vi "Rescale.vi"(8 "Error In":errorcluster, 11 "Pane Relief Main UI in":refnum<class "Pane Relief Main UI.lvclass">) -> (0 "Error Out":errorcluster, 3 "Pane Relief Main UI out":refnum<class "Pane Relief Main UI.lvclass">)   [LabVIEW 2017, in "Pane Relief Main UI.lvlib" / "Pane Relief Main UI.lvclass"]
uses:
  Pane Relief Main UI.lvclass
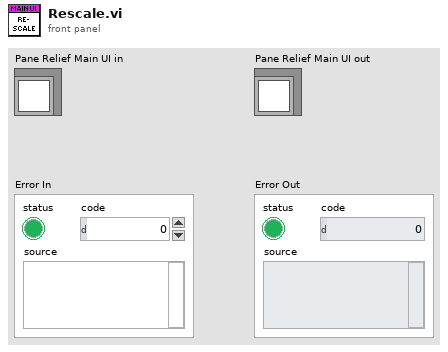
[diagram p1: front panel]
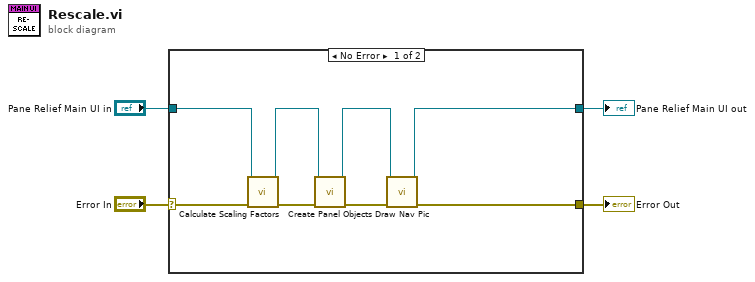
[diagram p0: block diagram]
diagram:
  n1 = case shown="No Error" "Error In" {
    selector: "Error In" -> [w8 w14]
    tunnel: [w5 w14] -> w1
    tunnel: [w7 w13] -> w3
    tunnel: "Pane Relief Main UI in" -> [w6 w13]
    frame No Error {
      n2 = call "Calculate Scaling Factors.vi"("error in (no error)"=w8, "Pane Relief Main UI in"=w6) -> ("error out"=w11:errorcluster, "Pane Relief Main UI out"=w12:refnum<class "Pane Relief Main UI.lvclass">)  [unwired: 8 in]
      n3 = call-dynamic "Create Panel Objects.vi"("Error In"=w11, "Pane Relief Main UI in"=w12) -> ("Error Out"=w9:errorcluster, "Pane Relief Main UI out"=w10:refnum<class "Pane Relief Main UI.lvclass">)  [unwired: 8 in]
      n4 = call-dynamic "Draw Nav Pic.vi"("Error In"=w9, "Pane Relief Main UI in"=w10) -> ("Error Out"=w5:errorcluster, "Pane Relief Main UI out"=w7:refnum<class "Pane Relief Main UI.lvclass">)  [unwired: 8 in]
    }
    frame Error {
    }
  }
  "Pane Relief Main UI out" <- w3
  "Error Out" <- w1
